vi "Draw Border.vi"(8 "error in (no error)":errorcluster, 11 "Rectangle Border in":refnum<class "Rectangle Border.lvclass">) -> (0 "error out":errorcluster, 2 "Border out":picture, 3 "Rectangle Border out":refnum<class "Rectangle Border.lvclass">)   [LabVIEW 2015, in "Rectangle Border.lvclass"]
uses:
  Rectangle Border.lvclass
  Rectangle Border.lvclass/Rectangle Border.ctl
  Scalable Border/Scalable Border.lvclass/Scalable Border.ctl
  Scalable Border/Scalable Border.lvclass
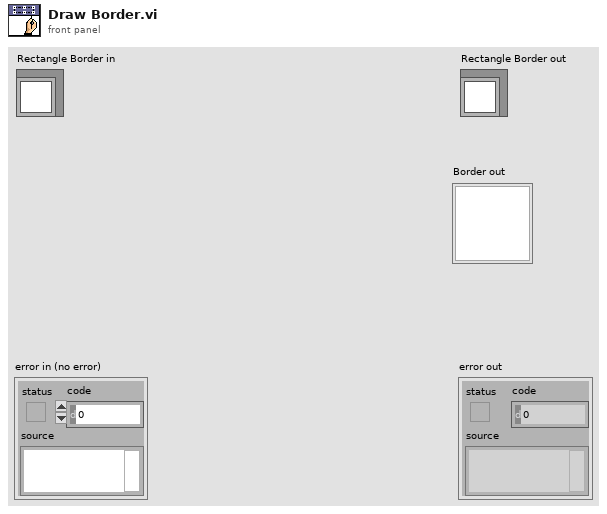
[diagram p1: front panel]
types:
  T1 = cluster{"left":i16, "top":i16, "right":i16, "bottom":i16}
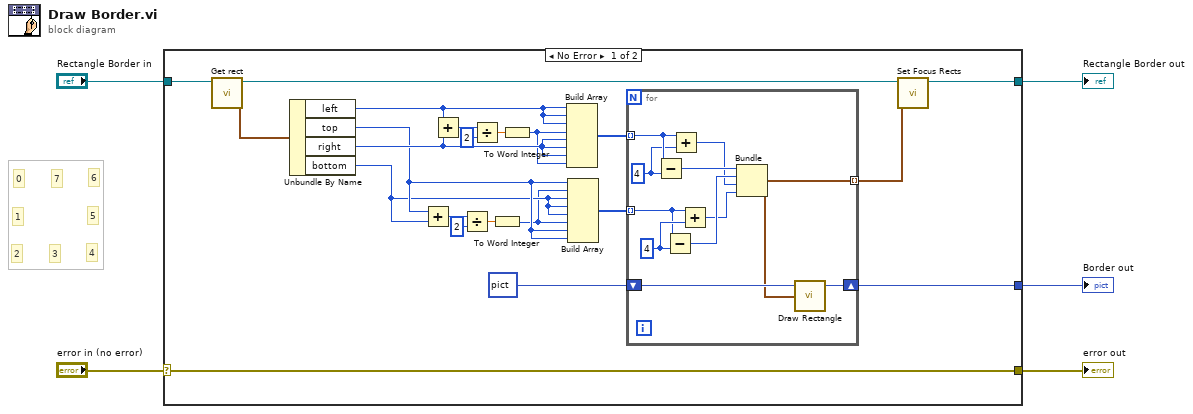
[diagram p0: block diagram]
diagram:
  # "4"
  # "5"
  # "6"
  # "3"
  # "7"
  # "2"
  # "1"
  # "0"
  n1 = case shown="No Error" "error in (no error)" {
    selector: "error in (no error)" -> [w27 w40]
    tunnel: "Rectangle Border in" -> [w11 w39]
    tunnel: [w12 _] -> w3
    tunnel: [w27 w40] -> w2
    tunnel: [w7 w39] -> w1
    frame No Error {
      n2 = call "Get rect.vi"("Rectangle Border in"=w11) -> ("rect"=w9:T1, "Rectangle Border out"=w10:refnum<class "Rectangle Border.lvclass">)  [unwired: 8 in, 1 out]
      n3 = Unbundle By Name(w9) -> ("left"=w26:i16, "top"=w17:i16, "right"=w25:i16, "bottom"=w16:i16)
      n4 = Add(x=w17, y=w16) -> (x+y=w18:i16)
      n5 = Add(x=w26, y=w25) -> (x+y=w24:i16)
      n6 = Divide(x=w18, y=i16 2) -> (x/y=w20:dbl)
      n7 = Divide(x=w24, y=i16 2) -> (x/y=w22:dbl)
      n8 = To Word Integer(number=w20) -> (16bit integer=w15:i16)
      n9 = To Word Integer(number=w22) -> (16bit integer=w21:i16)
      n10 = Build Array(w26, w26, w26, w21, w25, w25, w25, w21) -> (w14:i16[])
      n11 = Build Array(w17, w15, w16, w16, w16, w15, w17, w17) -> (w13:i16[])
      n12 = for {
        tunnel: w14 -> [w37] mode=indexing
        tunnel: w13 -> [w34] mode=indexing
        shift-right: [w29] -> w12
        shift-left: picture data[5B] ("new picture") -> [w38]
        tunnel: [w28] -> w6 mode=indexing
        w35 = i16 4 ("y")
        w36 = i16 4 ("y")
        n13 = Subtract(x=w37, y=w36) -> (x-y=w33:i16)
        n14 = Subtract(x=w34, y=w35) -> (x-y=w32:i16)
        n15 = Add(x=w37, y=w36) -> (x+y=w31:i16)
        n16 = Add(x=w34, y=w35) -> (x+y=w30:i16)
        n17 = Bundle(w33, w32, w31, w30) -> (w28:cluster{i16, i16, i16, i16})  [unwired: 1 in]
        n18 = call <vilib>:"Draw Rectangle.vi"("picture"=w38, "rect"=w28) -> ("new picture"=w29:picture)  [unwired: 7 in]
      }
      n19 = call "Set Focus Rects.vi"("Focus Rects"=w6, "Scalable Border in"=w10) -> ("Scalable Border out"=w7:refnum<class "Rectangle Border.lvclass">)  [unwired: 8 in, 1 out]
    }
    frame Error {
    }
  }
  "error out" <- w2
  "Rectangle Border out" <- w1
  "Border out" <- w3
